vi "Connection State.vi"(8 "error in (no error)":errorcluster, 11 "TCPMessageAPI in":refnum<class "TCPMessageAPI.lvclass">) -> (0 "error out":errorcluster, 2 "Connected":T1=enum."Connected", 3 "TCPMessageAPI out":refnum<class "TCPMessageAPI.lvclass">)   [LabVIEW 2020, in "Vecto.lvlib" / "TCPMessageAPI.lvclass"]
uses:
  TCPMessageAPI.lvclass
  TCPMessageAPI.lvclass/TCPMessageAPI.ctl
  Connected Status.ctl
  Vecto.lvlib
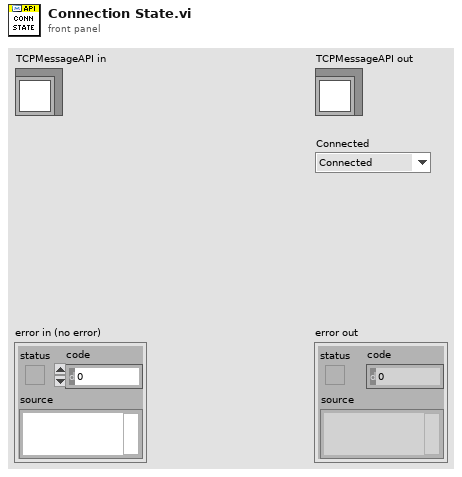
[diagram p1: front panel]
types:
  T1 = typedef "Vecto.lvlib/Connected Status.ctl" = enum16{"Disconnected", "Connected", "Bad Config", "Not Allowed", "Server"}
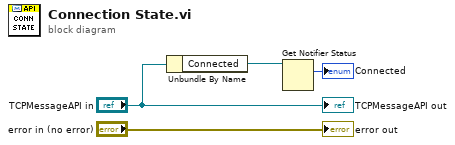
[diagram p0: block diagram]
diagram:
  n1 = Unbundle By Name("TCPMessageAPI in") -> ("Connected"=w2:refnum<notifier>)
  n2 = Get Notifier Status(notifier=w2) -> (current notification=→"Connected":T1)  [unwired: 1 in, 4 out]
  "error out" <- "error in (no error)"
  "TCPMessageAPI out" <- "TCPMessageAPI in"
